vi "YFM1-1.vi"() -> ()   [LabVIEW 2017]
uses:
  <vilib>/DAQmx/write.llb/DAQmx Write (Analog DBL 1Chan 1Samp).vi
  <vilib>/DAQmx/write.llb/DAQmx Write (Analog 1D DBL 1Chan NSamp).vi
  <vilib>/DAQmx/read.llb/DAQmx Read (Analog 1D DBL NChan 1Samp).vi
  <vilib>/DAQmx/create/channels.llb/DAQmx Create Channel (AO-Voltage-Basic).vi
  <vilib>/DAQmx/create/channels.llb/DAQmx Create Channel (AI-Voltage-Basic).vi
  <vilib>/DAQmx/configure/timing.llb/DAQmx Timing (Sample Clock).vi
  <vilib>/DAQmx/miscellaneous.llb/DAQmx Fill In Error Info.vi
  <vilib>/measure/NI_MABase.lvlib
  <vilib>/Analysis/NI_AALPro.lvlib
panel:
  out "Vg Array 2":dbl[](array[numeric])
  out "Numeric":dbl
  out "Array":dbl[](array[numeric])
  out "transfer characteristic":cluster{"Y":dbl[], "Y":dbl[]}(graph)
  out "error out 2":errorcluster
  out "gm":cluster{"dX/dt":dbl[], "Y":dbl[]}(graph)
  out "YFM":cluster{"Y":dbl[], dbl[]}(graph)
  out "theta":cluster{"X":dbl, "Y":dbl}[](graph)
  out "error out 3":errorcluster={"status"=TRUE, "code"=-200099, "source"="DAQmx Create Channel (AO-Voltage-Basic).vi:1870002<append>\n<B>Task Name: </B>_unnamedTask<0>"}
  out "error out":errorcluster={"status"=TRUE, "code"=-200477, "source"="YFM.vi<append>\n<B>Task Name: </B>_unnamedTask<1>"}
  out "Rct":dbl
  out "Vg Array":dbl[](array[numeric])
  in  "Start (V)":dbl=1.0
  in  "Stop (V)":dbl=2.0
  in  "Step":dbl=0.1
  out "# of step":dbl=nan
  in  "Vd":dbl
  in  "Id channels":tag="Dev9/ai0"
  in  "error in 2":errorcluster
  in  "Vg channels":tag="Dev3/ao0"
  in  "error in":errorcluster
  in  "Vd channels":tag="Dev3/ao1"
  in  "error in 3":errorcluster
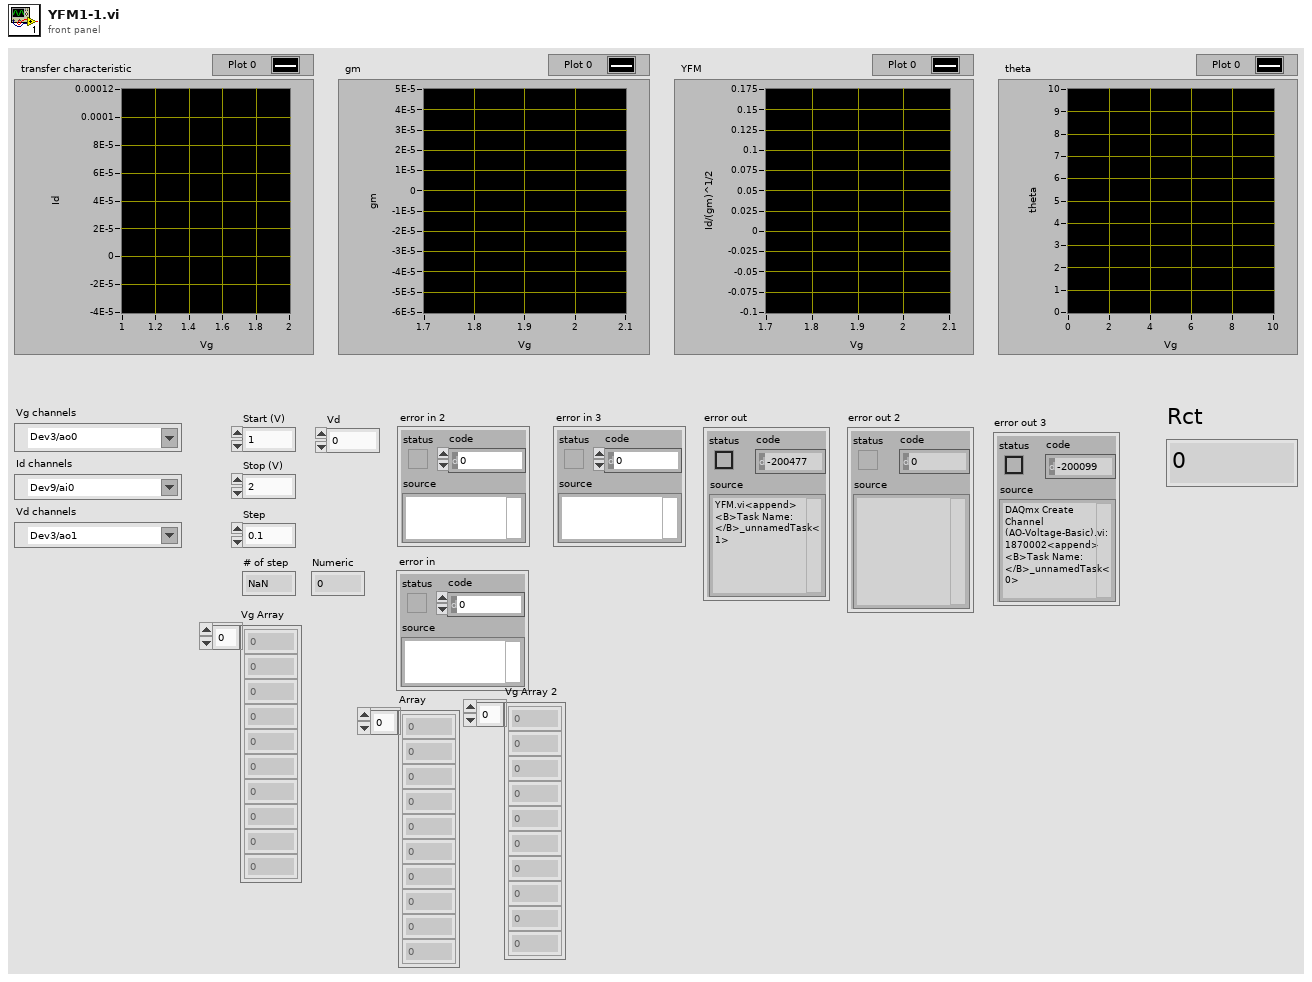
[diagram p1: front panel]
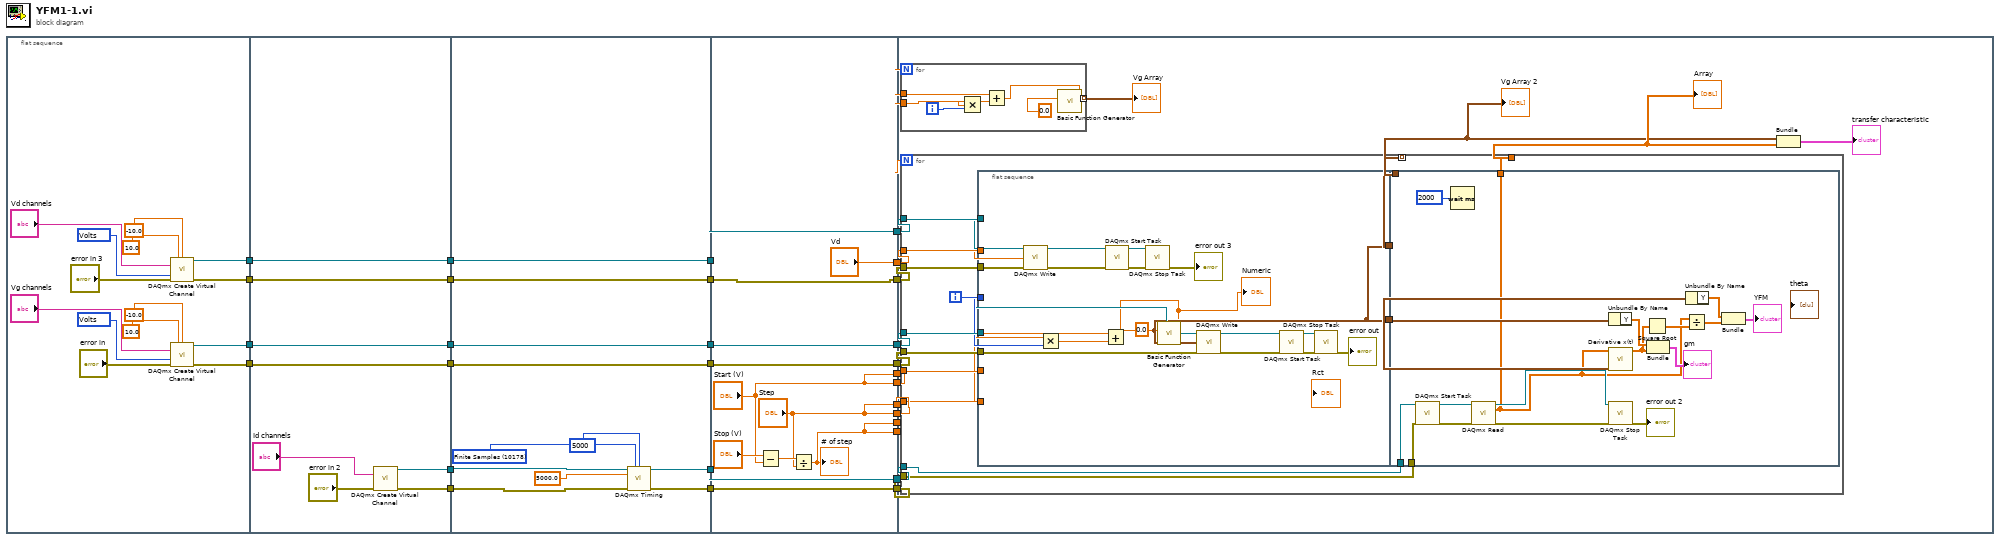
[diagram p0: block diagram]
diagram:
  n1 = flat-sequence {
    tunnel: [w38] -> w29
    tunnel: [w37] -> w28
    tunnel: [w32] -> w27
    tunnel: [w31] -> w26
    tunnel: w29 -> [w51]
    tunnel: [w51] -> w25
    tunnel: w28 -> [w50]
    tunnel: [w50] -> w24
    tunnel: [w47] -> w23
    tunnel: [w46] -> w22
    tunnel: [w45] -> w21
    tunnel: w27 -> [w45]
    tunnel: [w44] -> w20
    tunnel: w26 -> [w44]
    tunnel: w25 -> [w62]
    tunnel: w24 -> [w61]
    tunnel: w23 -> [w60]
    tunnel: w22 -> [w56]
    tunnel: [w62] -> w19
    tunnel: [w61] -> w18
    tunnel: [w55] -> w17
    tunnel: [w54] -> w16
    tunnel: [w53] -> w15
    tunnel: w21 -> [w53]
    tunnel: [w52] -> w14
    tunnel: w20 -> [w52]
    tunnel: w19 -> [w74]
    tunnel: w18 -> [w73]
    tunnel: w17 -> [w72]
    tunnel: w16 -> [w71]
    tunnel: [w74] -> w13
    tunnel: [w73] -> w12
    tunnel: [w72] -> w11
    tunnel: [w71] -> w10
    tunnel: ["Step"] -> w9
    tunnel: ["Start (V)"] -> w8
    tunnel: [w63] -> w7
    tunnel: ["Vd"] -> w6
    tunnel: [w67] -> w5
    tunnel: w15 -> [w67]
    tunnel: [w66] -> w4
    tunnel: w14 -> [w66]
    tunnel: ["Step"] -> w3
    tunnel: ["Start (V)"] -> w2
    tunnel: [w63] -> w1
    tunnel: w13 -> [w89]
    tunnel: w12 -> [w88]
    tunnel: w11 -> [w86]
    tunnel: w10 -> [w85]
    tunnel: w9 -> [w91]
    tunnel: w8 -> [w90]
    tunnel: w7 -> [w87]
    tunnel: w6 -> [w84]
    tunnel: w5 -> [w83]
    tunnel: w4 -> [w82]
    tunnel: w3 -> [w81]
    tunnel: w2 -> [w80]
    tunnel: w1 -> [w79]
    frame #0 {
      w34 = 10348 items=["Volts"=10348, "From Custom Scale"=10065] ("units")
      w39 = 10348 items=["Volts"=10348, "From Custom Scale"=10065] ("units")
      n2 = call-poly <vilib>:"DAQmx Create Virtual Channel.vi"("maximum value"=10.0, "minimum value"=-10.0, "physical channels"="Vd channels", "units"=w34, "error in"="error in 3") -> ("task out"=w32:refnum<k21>, "error out"=w31:errorcluster)  [unwired: 9 in]
      n3 = call-poly <vilib>:"DAQmx Create Virtual Channel.vi"("maximum value"=10.0, "minimum value"=-10.0, "physical channels"="Vg channels", "units"=w39, "error in"="error in") -> ("task out"=w38:refnum<k21>, "error out"=w37:errorcluster)  [unwired: 9 in]
    }
    frame #1 {
      n4 = call-poly <vilib>:"DAQmx Create Virtual Channel.vi"("physical channels"="Id channels", "error in"="error in 2") -> ("task out"=w47:refnum<k21>, "error out"=w46:errorcluster)  [unwired: 12 in]
    }
    frame #2 {
      w59 = 10178 items=["Finite Samples"=10178, "Continuous Samples"=10123, "Hardware Timed Single Point"=12522] ("sample mode")
      n5 = call-poly <vilib>:"DAQmx Timing.vi"("task/channels in"=w60, "sample mode"=w59, "samples per channel"=5000, "rate"=5000.0, "error in"=w56) -> ("task out"=w55:refnum<k21>, "error out"=w54:errorcluster)  [unwired: 9 in]
    }
    frame #3 {
      n6 = Subtract(x="Stop (V)", y="Start (V)") -> (x-y=w70:dbl)
      n7 = Divide(x=w70, y="Step") -> (x/y=w63:dbl)
      "# of step" <- w63
    }
    frame #4 {
      n8 = for {
        N: w79 -> [_]
        tunnel: w81 -> [w96]
        tunnel: w80 -> [w95]
        tunnel: [w92] -> w78 mode=indexing
        i -> [w97]
        n9 = Multiply(x=w96, y=w97) -> (x*y=w98:dbl)
        n10 = Add(x=w95, y=w98) -> (x+y=w94:dbl)
        n11 = call <vilib>:"Basic Function Generator.vi"("offset"=w94, "amplitude"=0.0) -> ("signal out"=w92:waveform(dbl))  [unwired: 7 in, 2 out]
      }
      "Vg Array" <- w78
      n12 = for {
        N: w87 -> [_]
        tunnel: w91 -> [w111]
        tunnel: w90 -> [w110]
        tunnel: w89 -> [w109]
        tunnel: w88 -> [w102]
        tunnel: w86 -> [w108]
        tunnel: w85 -> [w107]
        tunnel: w84 -> [w106]
        tunnel: w83 -> [w105]
        tunnel: w82 -> [w104]
        tunnel: [w100] -> w76
        tunnel: [w99] -> w75 mode=indexing
        i -> [w112]
        n13 = flat-sequence {
          tunnel: w112 -> [w131]
          tunnel: w111 -> [w130]
          tunnel: w110 -> [w129]
          tunnel: w109 -> [w128]
          tunnel: w106 -> [w127]
          tunnel: w105 -> [w124]
          tunnel: w104 -> [w123]
          tunnel: [w114] -> w103
          tunnel: w102 -> [w116]
          tunnel: [w114] -> w101
          tunnel: w108 -> [w150]
          tunnel: w107 -> [w149]
          tunnel: w103 -> [w137]
          tunnel: w101 -> [w135]
          tunnel: [w136] -> w100
          tunnel: [w135] -> w99
          frame #0 {
            n14 = call-poly <vilib>:"DAQmx Write.vi"("task/channels in"=w124, "data"=w127, "error in"=w123) -> ("task out"=w126:refnum<k21>, "error out"=w122:errorcluster)  [unwired: 10 in, 1 out]
            n15 = Multiply(x=w130, y=w131) -> (x*y=w134:dbl)
            n16 = Add(x=w129, y=w134) -> (x+y=w113:dbl)
            "Numeric" <- w113
            n17 = call <vilib>:"DAQmx Start Task.vi"("task/channels in"=w126, "error in"=w122) -> ("task out"=w125:refnum<k21>, "error out"=w121:errorcluster)  [unwired: 12 in]
            n18 = call <vilib>:"DAQmx Stop Task.vi"("task/channels in"=w125, "error in"=w121) -> ("error out"=→"error out 3":errorcluster)  [unwired: 12 in, 1 out]
            n19 = call <vilib>:"Basic Function Generator.vi"("offset"=w113, "amplitude"=0.0) -> ("signal out"=w114:waveform(dbl))  [unwired: 7 in, 2 out]
            n20 = call-poly <vilib>:"DAQmx Write.vi"("task/channels in"=w128, "data"=w114, "error in"=w116) -> ("task out"=w133:refnum<k21>, "error out"=w132:errorcluster)  [unwired: 10 in, 1 out]
            n21 = call <vilib>:"DAQmx Start Task.vi"("task/channels in"=w133, "error in"=w132) -> ("task out"=w119:refnum<k21>, "error out"=w118:errorcluster)  [unwired: 12 in]
            n22 = call <vilib>:"DAQmx Stop Task.vi"("task/channels in"=w119, "error in"=w118) -> ("error out"=→"error out":errorcluster)  [unwired: 12 in, 1 out]
          }
          frame #1 {
            n23 = call <vilib>:"DAQmx Start Task.vi"("task/channels in"=w150, "error in"=w149) -> ("task out"=w152:refnum<k21>, "error out"=w151:errorcluster)  [unwired: 12 in]
            n24 = Wait (ms)(milliseconds to wait=u32 2000) -> ()  [unwired: 1 out]
            n25 = call-poly <vilib>:"DAQmx Read.vi"("task/channels in"=w152, "error in"=w151) -> ("task out"=w147:refnum<k21>, "data"=w136:dbl[], "error out"=w146:errorcluster)  [unwired: 11 in]
            n26 = Unbundle By Name(w137) -> ("Y"=w143:dbl[])
            n27 = call <vilib>:"Derivative x(t).vi"("dt"=w137, "X"=w136) -> ("dX/dt"=w142:dbl[])  [unwired: 8 in, 1 out]
            n28 = call <vilib>:"DAQmx Stop Task.vi"("task/channels in"=w147, "error in"=w146) -> ("error out"=→"error out 2":errorcluster)  [unwired: 12 in, 1 out]
            n29 = Square Root(x=w142) -> (sqrt(x)=w141:dbl[])
            n30 = Bundle("Y"=w143, "dX/dt"=w142) -> (→"gm":cluster{"Y":dbl[], "dX/dt":dbl[]})  [unwired: 1 in]
            n31 = Divide(x=w136, y=w141) -> (x/y=w140:dbl[])
            n32 = Unbundle By Name(w137) -> ("Y"=w138:dbl[])
            n33 = Bundle("Y"=w138, w140) -> (→"YFM":cluster{"Y":dbl[], dbl[]})  [unwired: 1 in]
          }
        }
      }
      "Array" <- w76
      "Vg Array 2" <- w75
      n34 = Bundle(w75, "data"=w76) -> (→"transfer characteristic":cluster{waveform(dbl)[], "data":dbl[]})  [unwired: 1 in]
    }
  }
